vi "1.vi"() -> ()   [LabVIEW 2015]
uses:
  <vilib>/Analysis/NI_AALBase.lvlib
panel:
  out "Sine":dbl
  in  "Numeric":i32
  out "Error Out":errorcluster
  in  "Error In":errorcluster
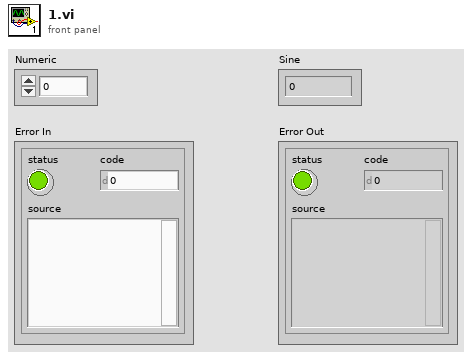
[diagram p1: front panel]
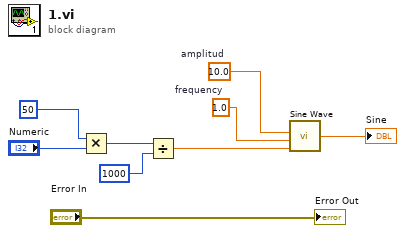
[diagram p0: block diagram]
diagram:
  w5 = 1.0  # frequency
  w6 = 10.0  # amplitud
  n1 = Multiply(x=50, y="Numeric") -> (x*y=w8:i32)
  n2 = Divide(x=w8, y=1000) -> (x/y=w4:dbl)
  n3 = call <vilib>:"Sine Wave.vi"("amplitude"=w6, "frequency"=w5, "phase in"=w4) -> ("phase out"=→"Sine":dbl)  [unwired: 2 in, 2 out]
  "Error Out" <- "Error In"
